vi "Yuzde30Kontrol.vi"(9 "Kahve":dbl(slide) scale=0.0..100.0, 10 "Çay":dbl(slide) scale=0.0..100.0, 11 "Su":dbl(slide) scale=0.0..100.0) -> (2 "Disabled":T1(ring))   [LabVIEW 2021]
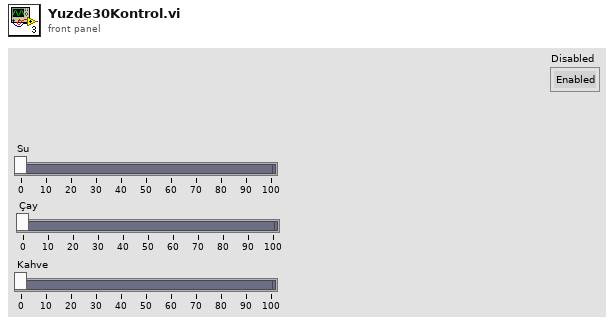
[diagram p1: front panel]
types:
  T1 = enum8{"Enabled", "Disabled", "Disabled and Grayed Out"}
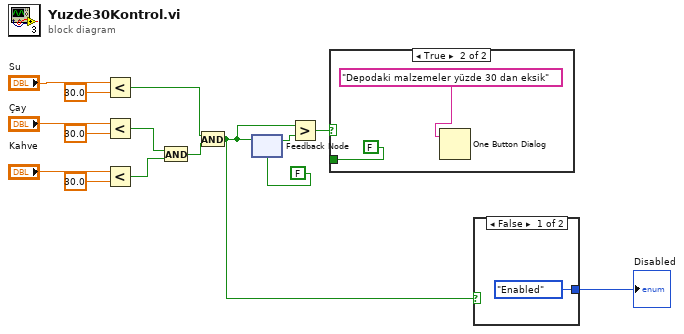
[diagram p0: block diagram]
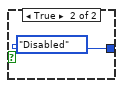
[diagram p2: hidden frame]
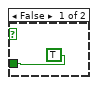
[diagram p3: hidden frame]
diagram:
  n1 = Less?(x="Su", y=30.0) -> (x < y?=w6:bool)
  n2 = Less?(x="Çay", y=30.0) -> (x < y?=w9:bool)
  n3 = Less?(x="Kahve", y=30.0) -> (x < y?=w8:bool)
  n4 = And(x=w9, y=w8) -> (x .and. y?=w7:bool)
  n5 = And(x=w6, y=w7) -> (x .and. y?=w1:bool)
  n6 = feedback-in #1(w1) -> ()
  n7 = feedback #1(FALSE) -> (w3:bool)
  n8 = Greater?(x=w1, y=w3) -> (0:w4:bool)
  n9 = case shown="True" w4 {
    tunnel: [TRUE FALSE] -> _
    frame False {
    }
    frame True {
      n10 = One Button Dialog(message="Depodaki malzemeler yüzde 30 dan eksik") -> ()  [unwired: 1 in, 1 out]
    }
  }
  n11 = case shown="False" w1 {
    tunnel: [T1."Enabled" ("Disabled") T1."Disabled" ("Disabled")] -> w2
    frame False {
    }
    frame True {
    }
  }
  "Disabled" <- w2
